vi "asi_set_backslash.vi"(4 "COM response delay":u32, 6 "Z backlash (um)":dbl=40.0 min=0.0 max=200.0 step=0.5, 8 "error in (no error)":errorcluster, 9 "Y backlash (um)":dbl min=0.0 max=200.0 step=0.5, 10 "X backlash (um)":dbl min=0.0 max=200.0 step=0.5, 11 "ASI Stage Port":refnum<visa-resource-name>) -> (0 "error out":errorcluster, 1 "RESPONSE":string, 2 "CMD":string)   [LabVIEW 2016]
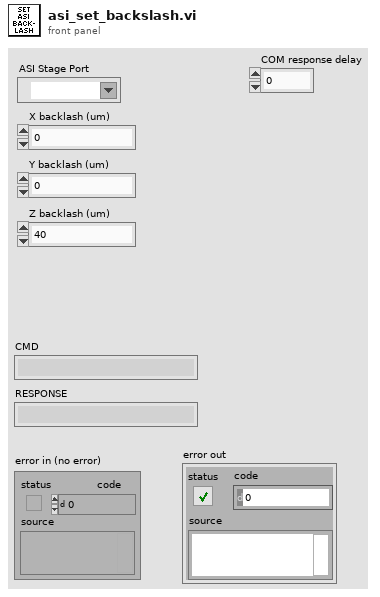
[diagram p1: front panel]
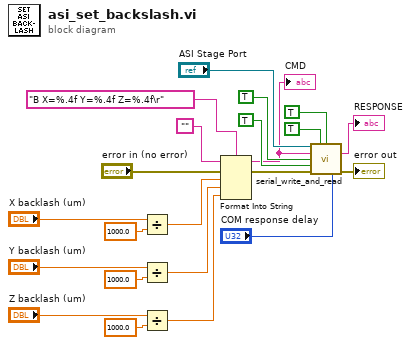
[diagram p0: block diagram]
diagram:
  n1 = Divide(x="X backlash (um)", y=1000.0) -> (x/y=w12:dbl)
  n2 = Divide(x="Y backlash (um)", y=1000.0) -> (x/y=w13:dbl)
  n3 = Divide(x="Z backlash (um)", y=1000.0) -> (x/y=w14:dbl)
  n4 = Format Into String(format string="B X=%.4f Y=%.4f Z=%.4f\r", initial string="", error in="error in (no error)", w12, w13, w14) -> (resulting string=w3:string, error out=w5:errorcluster)
  "CMD" <- w3
  n5 = call "serial_write_and_read.vi"("port name in"="ASI Stage Port", "reconnect?"=TRUE, "disconnect?"=TRUE, "write buffer"=w3, "do writing?"=TRUE, "expecting response?"=TRUE, "error in"=w5, "COM response delay"="COM response delay") -> ("read buffer"=→"RESPONSE":string, "error out"=→"error out":errorcluster)  [unwired: 5 in, 1 out]
